vi "LoadTestedLot.vi"(8 "error in (no error)":errorcluster, 11 "LotData in":refnum<class "LotData.lvclass">) -> (0 "error out":errorcluster, 3 "LotData out":refnum<class "LotData.lvclass">)   [LabVIEW 2012, in "LotData.lvclass"]
uses:
  LotData.lvclass
panel:
  in  "Wafer ID":string
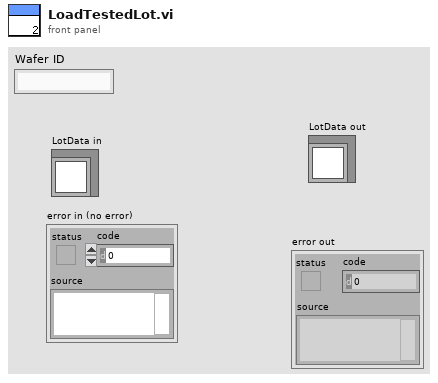
[diagram p1: front panel]
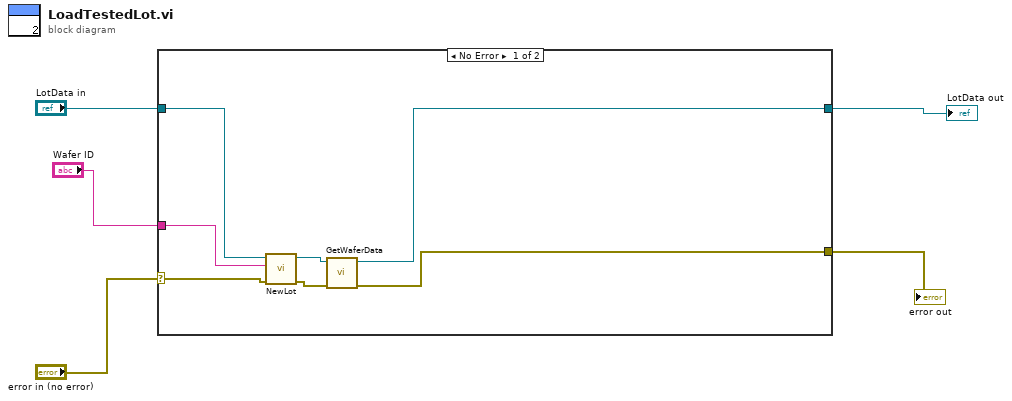
[diagram p0: block diagram]
diagram:
  n1 = case shown="No Error" "error in (no error)" {
    selector: "error in (no error)" -> [w9 w14]
    tunnel: [w7 w14] -> w4
    tunnel: [w8 w13] -> w2
    tunnel: "LotData in" -> [w10 w13]
    tunnel: "Wafer ID" -> [w6 _]
    frame No Error {
      n2 = call "NewLot.vi"("error in (no error)"=w9, "Wafer ID"=w6, "LotData in"=w10) -> ("error out"=w11:errorcluster, "LotData out"=w12:refnum<class "LotData.lvclass">)  [unwired: 7 in]
      n3 = call-dynamic "GetWaferData.vi"("error in (no error)"=w11, "LotData in"=w12) -> ("error out"=w7:errorcluster, "LotData out"=w8:refnum<class "LotData.lvclass">)  [unwired: 8 in]
    }
    frame Error {
    }
  }
  "error out" <- w4
  "LotData out" <- w2
